vi "6a.vi"(9 "U":dbl, 10 "f":dbl, 11 "A":dbl) -> (3 "Array":dbl[](array[numeric]))   [LabVIEW 2015]
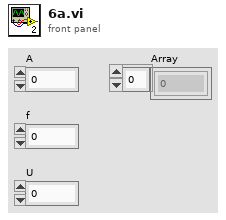
[diagram p1: front panel]
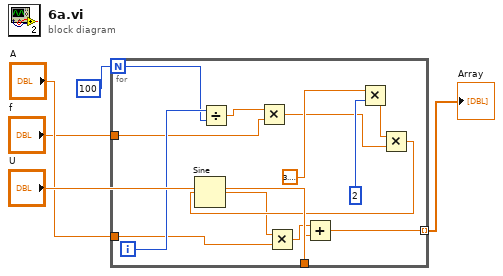
[diagram p0: block diagram]
diagram:
  n1 = for {
    N: 100 -> [w18]
    tunnel: "f" -> [w16]
    tunnel: "A" -> [w9]
    tunnel: "U" -> [w8]
    tunnel: [w6] -> w1 mode=indexing
    i -> [w19]
    n2 = Divide(x=w19, y=w18) -> (x/y=w17:dbl)
    n3 = Multiply(x=w17, y=w16) -> (x*y=w12:dbl)
    n4 = Multiply(x=3.141592653589793, y=2) -> (x*y=w13:dbl)
    n5 = Multiply(x=w13, y=w12) -> (x*y=w11:dbl)
    n6 = Sine(x=w11) -> (sin(x)=w10:dbl)
    n7 = Multiply(x=w10, y=w9) -> (x*y=w7:dbl)
    n8 = Add(x=w7, y=w8) -> (x+y=w6:dbl)
  }
  "Array" <- w1
